vi "Check Data Source.vi"(8 "error in (no error)":errorcluster, 9 "Argument":string, 10 "Current Path":path, 11 "Config":T1) -> (0 "error out":errorcluster, 3 "States":string)   [LabVIEW 2020, in "VI Properties Editor.lvlib"]
doc: "Checks if a certain data source within <B>Config</B> or <B>Current Path</B>, given by <B>Argument</B>, still exists, and enqueues the proper states after determining that."
uses:
  VI Properties Editor.lvlib
  CTLs/Config.ctl
  CTLs/Filter Info.ctl
  CTLs/Filter Column.ctl
  CTLs/Filter Type.ctl
  <vilib>/Utility/error.llb/Error Cluster From Error Code.vi
  <vilib>/ErrorRing/Error Ring.xnode
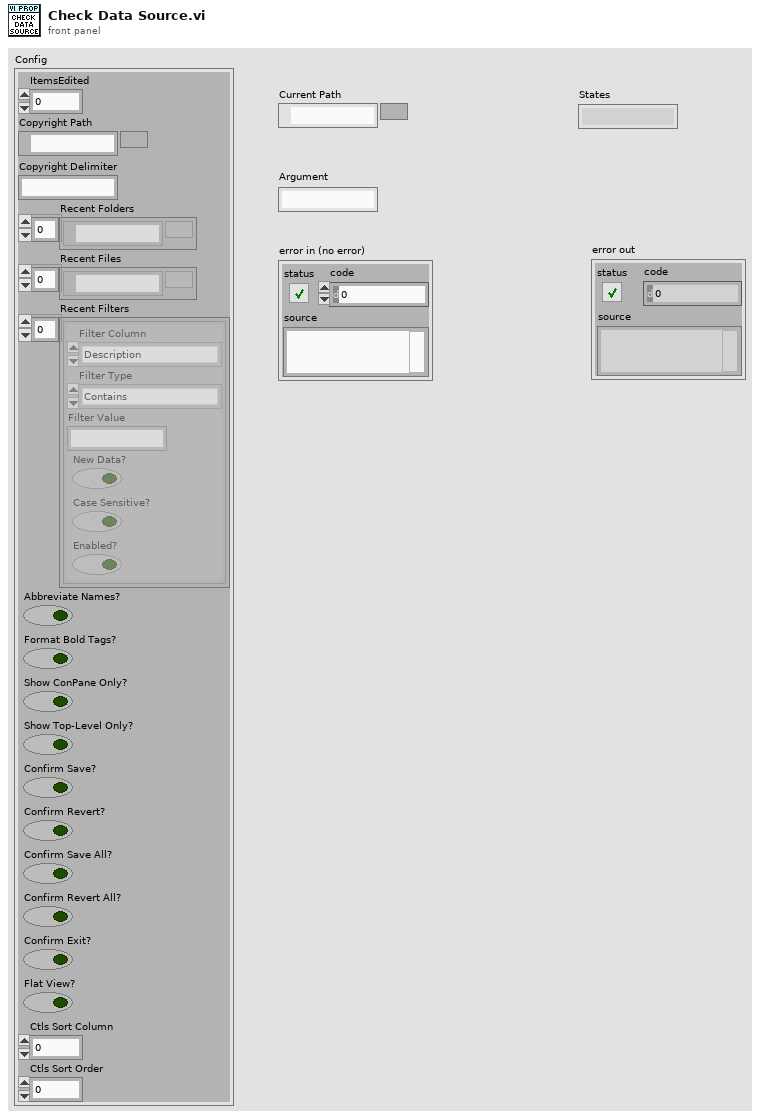
[diagram p1: front panel]
types:
  T1 = typedef "VI Properties Editor.lvlib/Config.ctl" = cluster{"ItemsEdited":u32, "Copyright Path":path, "Copyright Delimiter":string, "Recent Folders":path[], "Recent Files":path[], "Recent Filters":T2[], "Abbreviate Names?":bool, "Format Bold Tags?":bool, "Show ConPane Only?":bool, "Show Top-Level Only?":bool, "Confirm Save?":bool, "Confirm Revert?":bool, "Confirm Save All?":bool, "Confirm Revert All?":bool, "Confirm Exit?":bool, "Flat View?":bool, "Ctls Sort Column":i32, "Ctls Sort Order":i32}
  T2 = typedef "VI Properties Editor.lvlib/Filter Info.ctl" = cluster{"Filter Column":T3, "Filter Type":T4, "Filter Value":string, "New Data?":bool, "Case Sensitive?":bool, "Enabled?":bool}
  T3 = typedef "VI Properties Editor.lvlib/Filter Column.ctl" = enum16{"Name", "Path", "Type", "Window Title", "Description", "Help Path", "Help Tag", "Custom Title?", "Reentrancy", "Inlined?", "Help URL", "Help Type", "Allow Debugging?", "Auto Error Handling?", "Run When Opened?", "Suspend When Called?", "Priority", "Preferred Exec Sytem", "Control Label", "Control Caption", "Control Description", "Control Tip Strip"}
  T4 = typedef "VI Properties Editor.lvlib/Filter Type.ctl" = enum16{"Contains", "Equals", "Starts with", "Ends with", "Is empty", "Does not contain", "Does not equal", "Is not empty"}
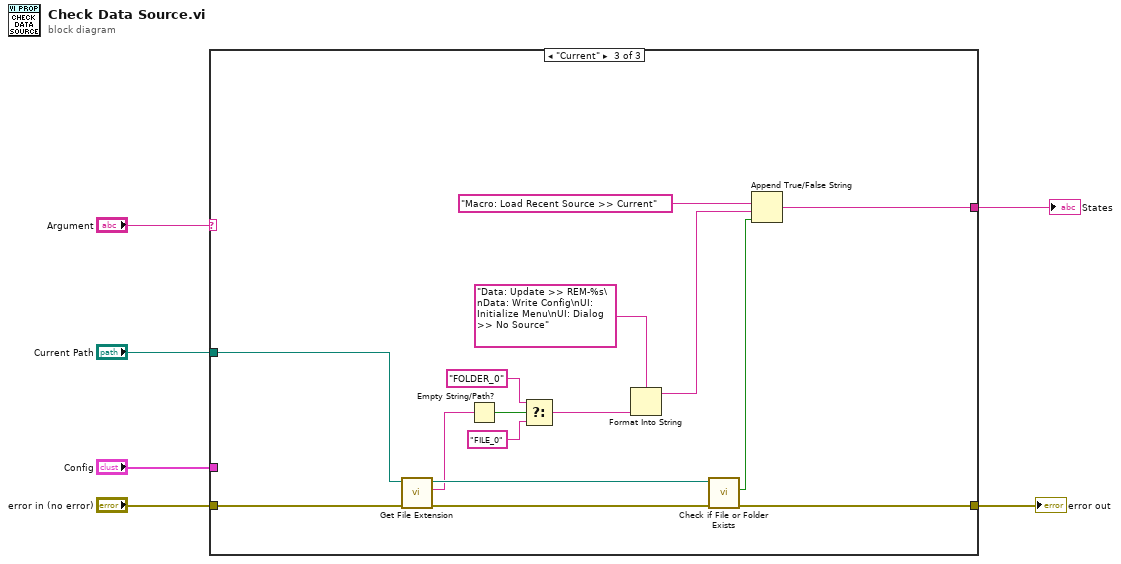
[diagram p0: block diagram]
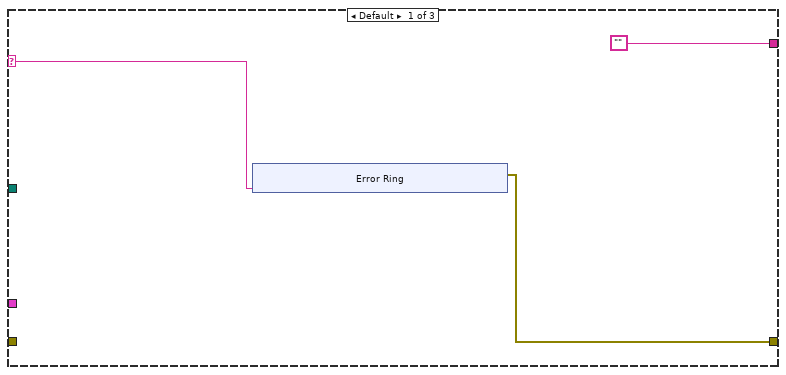
[diagram p2: hidden frame]
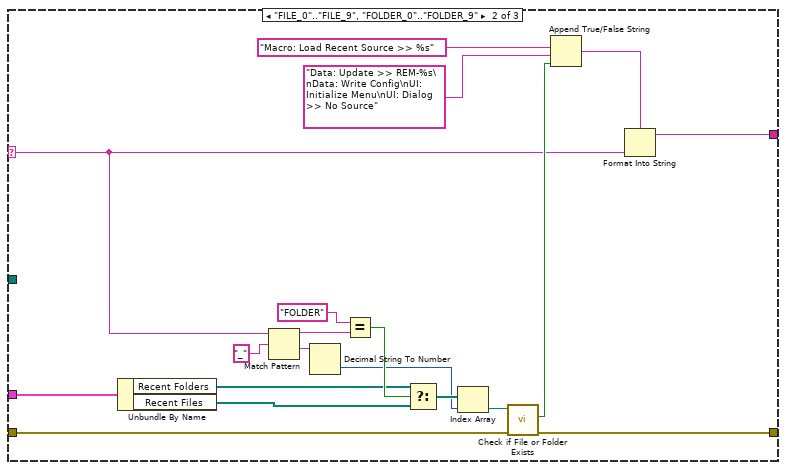
[diagram p3: hidden frame]
diagram:
  n1 = case shown="\"Current\"" "Argument" {
    selector: "Argument" -> [w9 w19 _]
    tunnel: "Config" -> [_ w21 _]
    tunnel: "error in (no error)" -> [_ w20 w47]
    tunnel: ["" w18 w36] -> w3
    tunnel: [w8 w17 w48] -> w2
    tunnel: "Current Path" -> [_ _ w46]
    frame Default {
      n2 = xnode "Error Ring"("parameter 0"=w9) -> ("error out"=w8:errorcluster)
    }
    frame "FILE_0".."FILE_9", "FOLDER_0".."FOLDER_9" {
      n3 = Unbundle By Name(w21) -> ("Recent Folders"=w30:path[], "Recent Files"=w29:path[])
      n4 = Match Pattern(string=w19, regular expression="_") -> (before substring=w33:string, after substring=w34:string)  [unwired: 1 in, 2 out]
      n5 = Decimal String To Number(string=w34) -> (number=w27:i32)  [unwired: 2 in, 1 out]
      n6 = Equal?(x="FOLDER", y=w33) -> (x = y?=w31:bool)
      n7 = Select(t=w30, s=w31, f=w29) -> (s? t:f=w28:path[])
      n8 = Index Array(array=w28, index=w27) -> (element=w26:path)
      n9 = call <vilib>:"Check if File or Folder Exists.vi"("error in (no error)"=w20, "path"=w26) -> ("error out"=w17:errorcluster, "file or folder exists?"=w25:bool)  [unwired: 7 in, 1 out]
      n10 = Append True/False String(1:w25, 2:"Data: Update >> REM-%s\nData: Write Config\nUI: Initialize Menu\nUI: Dialog >> No Source", 3:"Macro: Load Recent Source >> %s") -> (0:w22:string)  [unwired: 1 in]
      n11 = Format Into String(format string=w22, w19) -> (resulting string=w18:string)  [unwired: 2 in, 1 out]
    }
    frame "Current" {
      n12 = call <vilib>:"Get File Extension.vi"("error in (no error)"=w47, "file"=w46) -> ("error out"=w44:errorcluster, "lowercase file extension"=w43:string, "dup file"=w45:path)  [unwired: 5 in, 2 out]
      n13 = Empty String/Path?(string/path=w43) -> (empty?=w42:bool)
      n14 = Select(t="FOLDER_0", s=w42, f="FILE_0") -> (s? t:f=w38:string)
      n15 = Format Into String(format string="Data: Update >> REM-%s\nData: Write Config\nUI: Initialize Menu\nUI: Dialog >> No Source", w38) -> (resulting string=w37:string)  [unwired: 2 in, 1 out]
      n16 = call <vilib>:"Check if File or Folder Exists.vi"("error in (no error)"=w44, "path"=w45) -> ("error out"=w48:errorcluster, "file or folder exists?"=w50:bool)  [unwired: 7 in, 1 out]
      n17 = Append True/False String(1:w50, 2:w37, 3:"Macro: Load Recent Source >> Current") -> (0:w36:string)  [unwired: 1 in]
    }
  }
  "error out" <- w2
  "States" <- w3
